vi "Configure Curve Header.vi"(0 "VISA resource name":refnum<visa-resource-name>, 1 "Curve Data Format (1:mV/K)":u16(ring)=1 items=["mV/K"=1, "V/K"=2, "Ohms/K"=3, "Log Ohms/K"=4], 2 "Limit Value (375.000)":dbl=375.0 format="%.3f", 5 "Curve (21)":dbl=21.0, 7 "Curve Name (\"\")":string, 9 "Curve Serial Number (\"\")":string, 11 "error in (no error)":errorcluster, 12 "Coefficient (1:Negative)":u16(ring)=1 items=["Negative"=1, "Positive"=2]) -> (4 "VISA resource name out":refnum<visa-resource-name>, 15 "error out":errorcluster)   [LabVIEW 2012, in "Lake Shore 336.lvlib"]
doc: "This VI configures a curve header. Each curve has parameters that are used for identification and to allow the instrument to use the curve effectively. The parameters must be set correctly before a curve can be used for temperature conversion or tempersture control."
uses:
  Lake Shore 336.lvlib
  Instance           1 30Saved   Configure Curve Header .vi
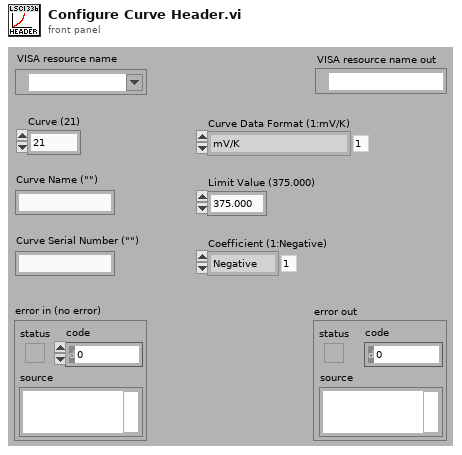
[diagram p1: front panel]
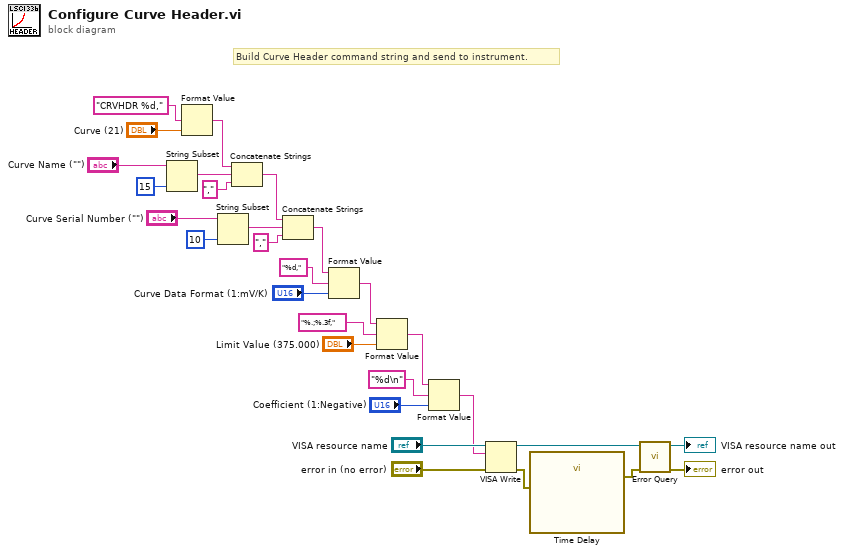
[diagram p0: block diagram]
diagram:
  # "Build Curve Header command string and send to instrument."
  n1 = String Subset(string="Curve Name (\"\")", length (rest)=15) -> (substring=w16:string)  [unwired: 1 in]
  n2 = Format Value(format string="CRVHDR %d,", value (0)="Curve (21)") -> (output string=w18:string)  [unwired: 1 in]
  n3 = String Subset(string="Curve Serial Number (\"\")", length (rest)=10) -> (substring=w14:string)  [unwired: 1 in]
  n4 = Concatenate Strings(w18, w16, ",") -> (w12:string)
  n5 = Concatenate Strings(w12, w14, ",") -> (w10:string)
  n6 = Format Value(string ("")=w10, format string="%d,", value (0)="Curve Data Format (1:mV/K)") -> (output string=w9:string)
  n7 = Format Value(string ("")=w9, format string="%.;%.3f,", value (0)="Limit Value (375.000)") -> (output string=w5:string)
  n8 = Format Value(string ("")=w5, format string="%d\n", value (0)="Coefficient (1:Negative)") -> (output string=w3:string)
  n9 = VISA Write(VISA resource name="VISA resource name", write buffer=w3, error in (no error)="error in (no error)") -> (VISA resource name out=w26:refnum<visa-resource-name>, error out=w8:errorcluster)  [unwired: 1 out]
  n10 = call "Time Delay"("error in (no error)"=w8) -> ("error out"=w7:errorcluster)  [unwired: 10 in]
  n11 = call "Error Query.vi"("error in (no error)"=w7, "VISA resource name"=w26) -> ("error out"=→"error out":errorcluster, "VISA resource name out"=→"VISA resource name out":refnum<visa-resource-name>)  [unwired: 7 in, 1 out]
